vi "CRC_A965 .vi"(11 "U8":u8[](array[numeric]) format="%.0x") -> (3 "CRC-16":u16 format="%.0x")   [LabVIEW 2021]
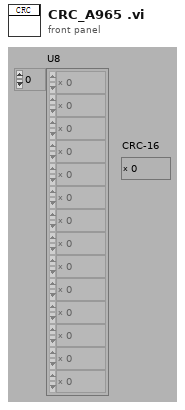
[diagram p1: front panel]
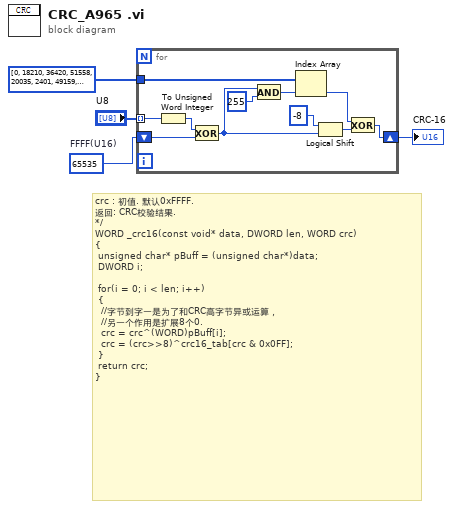
[diagram p0: block diagram]
diagram:
  w4 = u16 65535  # FFFF(U16)
  # "crc : 初值. 默认0xFFFF.\n返回: CRC校验结果.\n*/\nWORD _crc16(const void* data, DWORD len, WORD crc)\n{\n\tunsigned char* pBuff = (unsigned char*)data;\n\tDWORD i;\n\n\tfor(i = 0; i < len; i++)\n\t{\n\t\t//字节到字一是为了和CRC高字节异或运算，\n\t\t//另一个作用是扩展8个0.\n\t\tcrc = crc^(WORD)pBuff[i];\n\t\tcrc = (crc>>8)^crc16_tab[crc & 0x0FF];\n\t}\n\treturn crc;\n}"
  n1 = for {
    tunnel: "U8" -> [w14] mode=indexing
    tunnel: u16[] [0, 18210, 36420, 51558, 20035, 2401, 49159, 34597, 40070, 56228, 4802, 21984, 53957, 38375, 23681, 7075, 27591, 11493, 58755, 41633, 9604, 25254, 43968, 60642, 63297, 45155, 30981, 15911, 47362, 65056, 14150, 28772, 55182, 37036, 22986, 7912, 39373, 57071, 6025, 20651, 19208, 3114, 50508, 33390, 1355, 17001, 35599, 52269, 48201, 64363, 12813, 29999, 61962, 46376, 31822, 15212, 8399, 26605, 44683, 59817, 28300, 10670, 57544, 42986, 64983, 47861, 29587, 13489, 45972, 62646, 15824, 31474, 24913, 9843, 61205, 43063, 12050, 26672, 41302, 58996, 38416, 53554, 6228, 24438, 55379, 40817, 22039, 4405, 2710, 19892, 34002, 50160, 17621, 1015, 51857, 36275, 10841, 28027, 42013, 58175, 25626, 9016, 59998, 44412, 46815, 61949, 14491, 32697, 63644, 49086, 30424, 12794, 16798, 1724, 53210, 35064, 4061, 18687, 33177, 50875, 56600, 39482, 21340, 5246, 37723, 54393, 7455, 23101, 43365, 60999, 10017, 24579, 59174, 40964, 26978, 11840, 13795, 29377, 48039, 64645, 31648, 15490, 62948, 45766, 49826, 34176, 19686, 3012, 36065, 52163, 677, 17799, 24100, 6406, 53344, 38722, 4199, 22341, 40483, 55553, 32491, 14793, 61615, 46989, 12456, 30602, 48876, 63950, 57965, 42319, 27689, 11019, 44078, 60172, 8810, 25928, 5420, 21006, 39784, 56394, 23407, 7245, 54571, 37385, 35242, 52872, 2030, 16588, 51177, 32971, 18861, 3727, 21682, 5008, 56054, 40404, 6897, 24019, 38069, 54167, 51252, 36630, 18032, 338, 34423, 49493, 2099, 20241, 16245, 30807, 45361, 62995, 28982, 13844, 65394, 47184, 41971, 58577, 11703, 27285, 60848, 43666, 25588, 9430, 33596, 50206, 3448, 19034, 52607, 35421, 17211, 1049, 8122, 22680, 37374, 55004, 20985, 5851, 57277, 39071, 59643, 45017, 26303, 8605, 42680, 57754, 10492, 28638, 29821, 13151, 64057, 48411, 14910, 32028, 46202, 62296] ("数组") -> [w15]
    shift-right: [w6] -> w2
    shift-left: w4 -> [w11]
    n2 = To Unsigned Word Integer(number=w14) -> (unsigned 16bit integer=w13:u16)
    n3 = Exclusive Or(1:w11, 2:w13) -> (0:w5:u16)
    n4 = And(x=w5, y=u16 255) -> (x .and. y?=w9:u16)
    n5 = Index Array(array=w15, index=w9) -> (element=w10:u16)
    n6 = Logical Shift(y=i16 -8, x=w5) -> (x << y=w7:u16)
    n7 = Exclusive Or(1:w7, 2:w10) -> (0:w6:u16)
  }
  "CRC-16" <- w2
